vi "WaveFormGen.vi"(0 "电源干扰测试状态":refnum<vi>, 1 "开始测试":refnum<vi>, 2 "电池恢复波形参数":T4={"最低电压持续时间 2"=10, "最终电压 2"=12.0, "最低电压2"=7.5, "初始电压时间 2"=10, "初始电压2"=12.0, "恢复时间(s)"=600}, 5 "ACC点火波形参数":T5={"初始电压"=12.0, "初始电压时间"=500, "最低点电压"=7.5, "上升点电压"=10.0, "从最低点到上升点时间"=100.0, "波动电压持续时间"=200, "从上升点到最终点时间"=3000.0, "最终点电压"=12.0, "最低点持续时间"=20} {"从上升点到最终点时间" format="%#_13g"; "从最低点到上升点时间" format="%#_13g"}, 7 "电压瞬断波形参数":cluster{"电源电压":dbl, "周期(ms)":i32, "周期数":i32}={"电源电压"=14.0, "周期(ms)"=2, "周期数"=2} {"电源电压" format="%#_13g"}, 9 "电压缓变波形参数":T3={"最低电压持续时间 3"=1, "最高电压 3"=12.0, "最低电压2 2"=5.0, "初始电压时间 3"=1, "初始电压2 2"=12.0, "变化档位"=enum."1V/s", "周期数"=10}, 12 "+B电压开机参数":cluster{"+B电压":dbl, "持续时间(s)":i32}={"+B电压"=12.3, "持续时间(s)"=1} {"+B电压" format="%#_13g"}, 13 "测试项目":T1(ring), 14 "电源正弦纹波参数":T2={"频率1"=500.0, "幅度Vp"=4.0, "频率2"=20000.0, "频率3"=500.0, "电压Vs"=14.0, "周期数 3"=1} {"电压Vs" format="%#_13g"; "频率3" format="%#_13g"; "频率2" format="%#_13g"; "幅度Vp" format="%#_13g"; "频率1" format="%#_13g"}) -> (4 "waveform out":waveform(dbl))   [LabVIEW 2013]
uses:
  <vilib>/Analysis/1siggen.llb/Ramp Pattern by Samples.vi
  <vilib>/Waveform/WDTOps.llb/WDT Append Waveforms DBL.vi
  <vilib>/Analysis/NI_AALBase.lvlib
  <vilib>/measure/NI_MABase.lvlib
panel:
  # "(ms)"
  # "(ms)"
  # "(ms)"
  # "(ms)"
  # "(ms)"
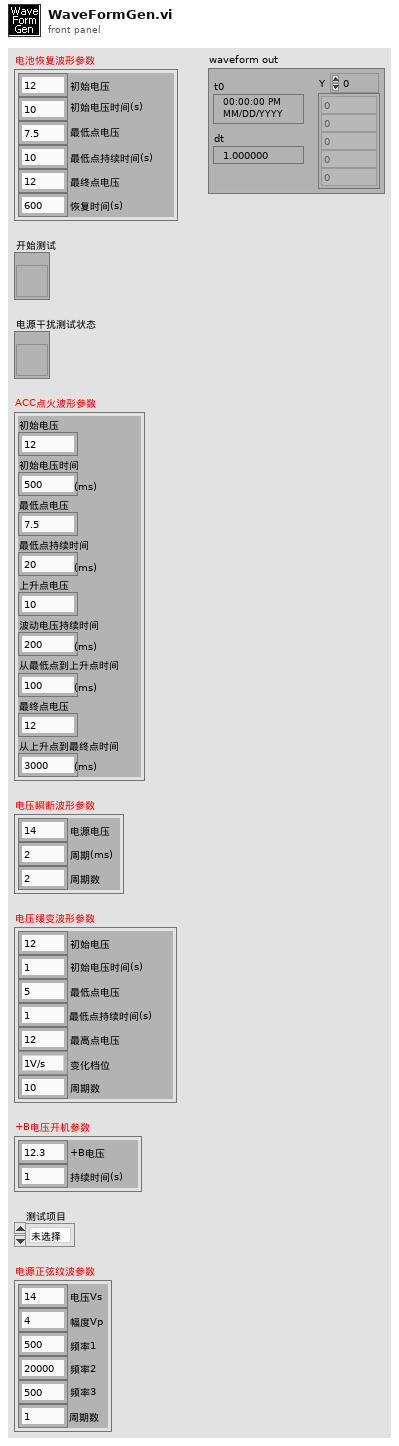
[diagram p1: front panel]
types:
  T1 = enum32{"未选择", "电源正弦纹波", "电压瞬断", "电池恢复", "电压缓变", "+B电压开机", "ACC点火"}
  T2 = cluster{"频率1":dbl, "幅度Vp":dbl, "频率2":dbl, "频率3":dbl, "电压Vs":dbl, "周期数 3":i32}
  T3 = cluster{"最低电压持续时间 3":i32, "最高电压 3":dbl, "最低电压2 2":dbl, "初始电压时间 3":i32, "初始电压2 2":dbl, "变化档位":enum16{"1V/s", "10V/s", "1V/min"}, "周期数":i32}
  T4 = cluster{"最低电压持续时间 2":i32, "最终电压 2":dbl, "最低电压2":dbl, "初始电压时间 2":i32, "初始电压2":dbl, "恢复时间(s)":i32}
  T5 = cluster{"初始电压":dbl, "初始电压时间":i32, "最低点电压":dbl, "上升点电压":dbl, "从最低点到上升点时间":dbl, "波动电压持续时间":i32, "从上升点到最终点时间":dbl, "最终点电压":dbl, "最低点持续时间":i32}
  T6 = enum8{"Enabled", "Disabled", "Disabled and Grayed Out"}
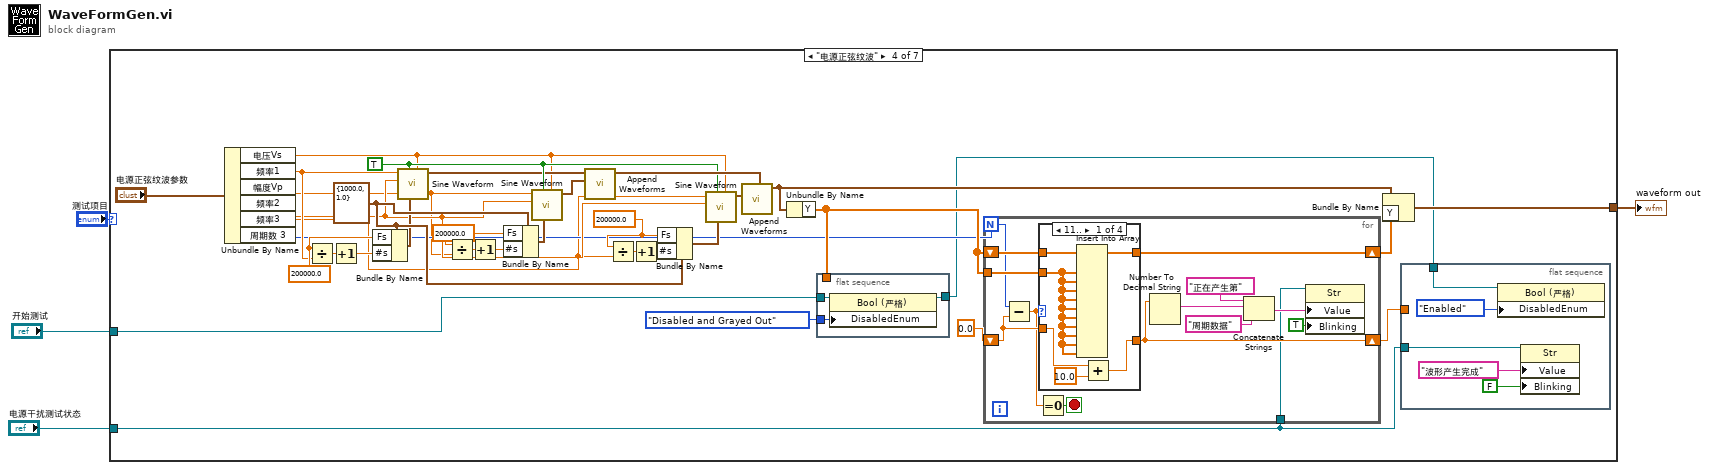
[diagram p0: block diagram]
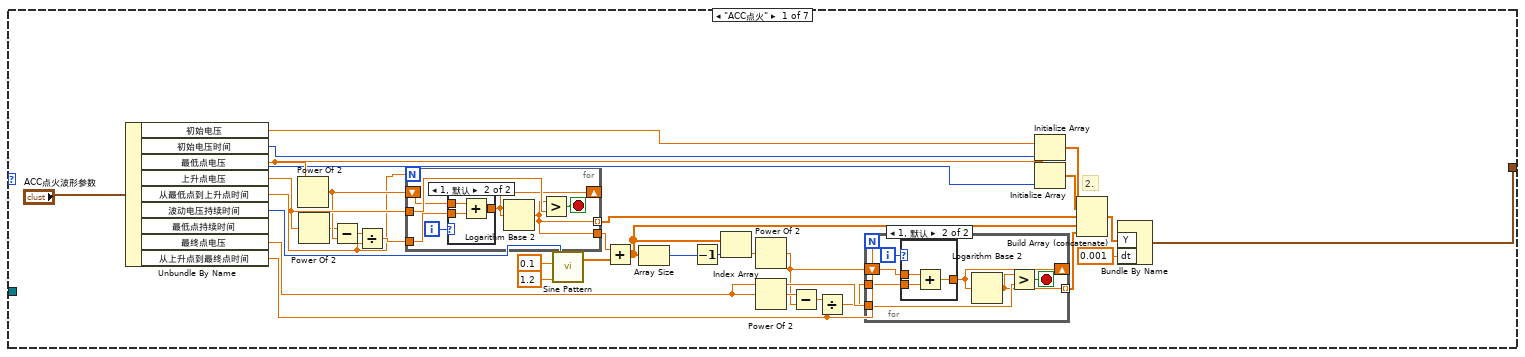
[diagram p2: hidden frame]
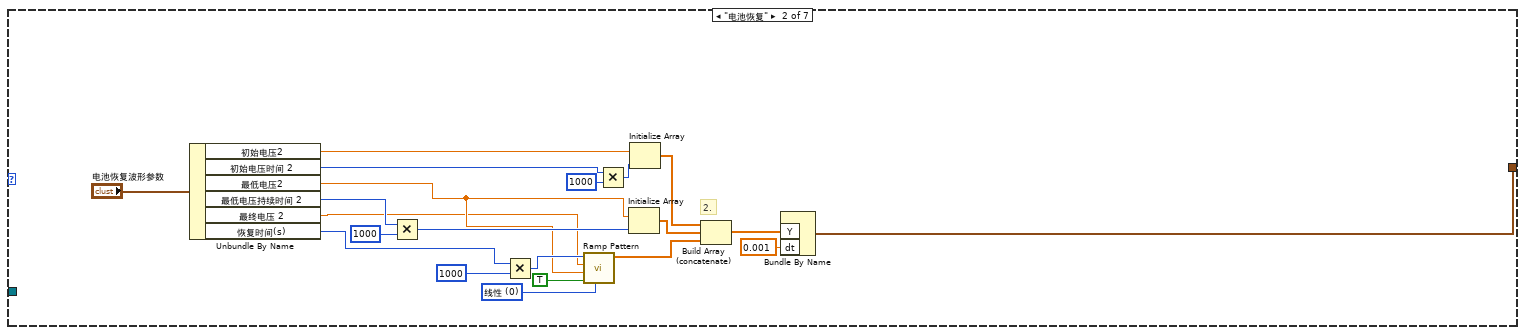
[diagram p5: hidden frame]
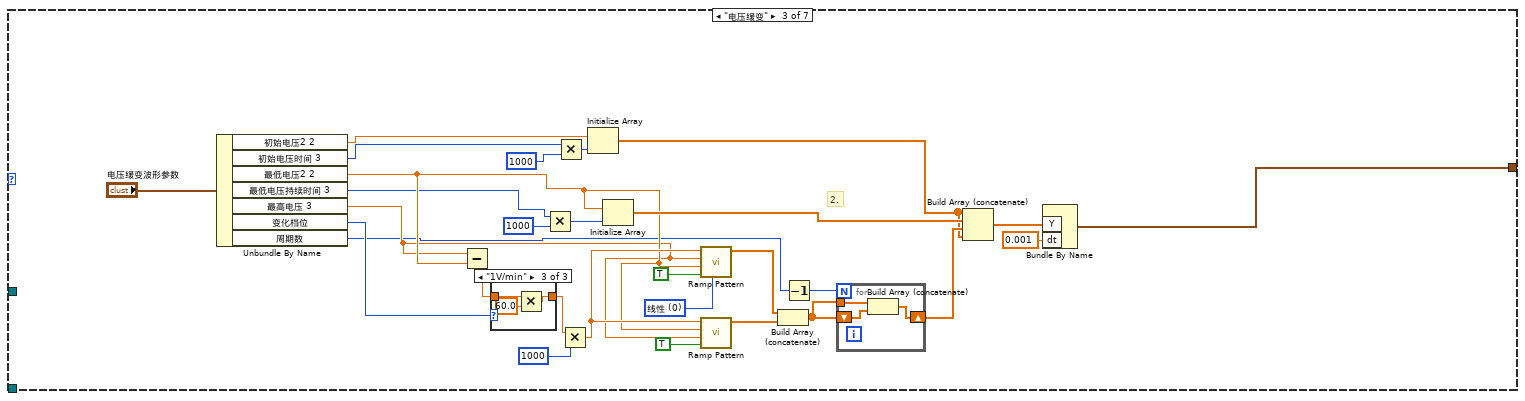
[diagram p6: hidden frame]
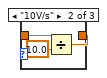
[diagram p8: hidden frame]
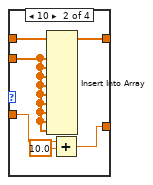
[diagram p9: hidden frame]
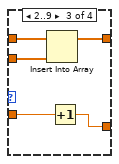
[diagram p10: hidden frame]
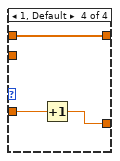
[diagram p11: hidden frame]
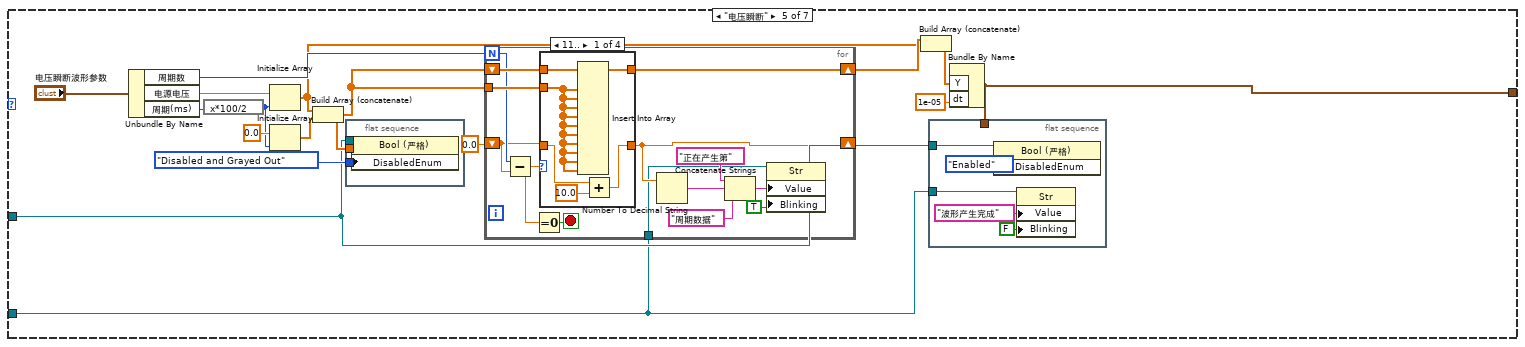
[diagram p12: hidden frame]
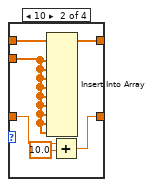
[diagram p13: hidden frame]
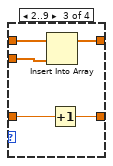
[diagram p14: hidden frame]
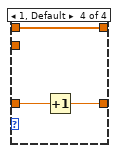
[diagram p15: hidden frame]
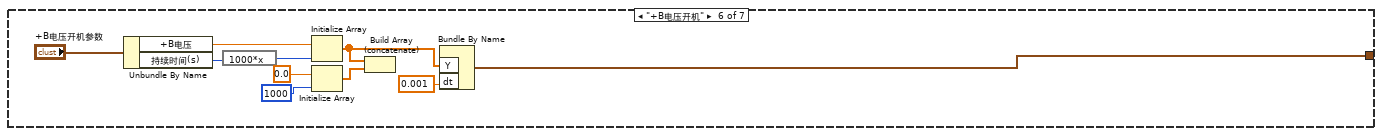
[diagram p16: hidden frame]
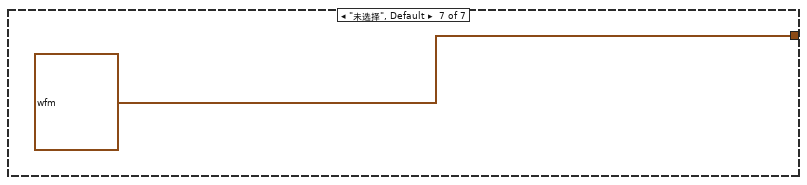
[diagram p17: hidden frame]
diagram:
  n1 = case shown="\"电源正弦纹波\"" "测试项目" {
    tunnel: [w10 w67 w90 w154 w199 w258 waveform(dbl) {"t0"=timestamp(0 s since 1904-01-01), "dt"=1.0, "Y"=[]} ("waveform out")] -> w3
    tunnel: "开始测试" -> [_ _ _ w122 w198 _ _]
    tunnel: "电源干扰测试状态" -> [_ _ _ w120 w197 _ _]
    frame "ACC点火" {
      # "2."
      n2 = Unbundle By Name("ACC点火波形参数") -> ("初始电压"=w34:dbl, "初始电压时间"=w6:i32, "最低点电压"=w35:dbl, "上升点电压"=w36:dbl, "从最低点到上升点时间"=w8:dbl, "波动电压持续时间"=w9:i32, "最低点持续时间"=w5:i32, "最终点电压"=w37:dbl, "从上升点到最终点时间"=w7:dbl)
      n3 = Power Of 2(x=w35) -> (2^x=w17:dbl)
      n4 = Power Of 2(x=w36) -> (2^x=w14:dbl)
      n5 = Subtract(x=w14, y=w17) -> (x-y=w15:dbl)
      n6 = Divide(x=w15, y=w8) -> (x/y=w16:dbl)
      n7 = for {
        N: w8 -> [_]
        tunnel: [w49] -> w32 mode=indexing
        tunnel: w36 -> [w54]
        shift-right: [w52] -> _
        shift-left: w17 -> [w53]
        tunnel: w16 -> [w51]
        tunnel: [w49] -> w30
        i -> [w50]
        stop <- w55 stop-if-true
        n8 = case shown="1, 默认" w50 {
          tunnel: w53 -> [w56 w59]
          tunnel: [w56 w58] -> w52
          tunnel: w51 -> [_ w57]
          frame 0 {
          }
          frame 1, Default {
            n9 = Add(x=w59, y=w57) -> (x+y=w58:dbl)
          }
        }
        n10 = Logarithm Base 2(1:w52) -> (0:w49:dbl)
        n11 = Greater?(x=w49, y=w54) -> (0:w55:bool)
      }
      n12 = call <vilib>:"Sine Pattern.vi"("cycles"=1.2, "amplitude"=0.1, "samples"=w9) -> ("Sinusoidal Pattern"=w24:dbl[])  [unwired: 1 in, 1 out]
      n13 = Add(x=w30, y=w24) -> (x+y=w29:dbl[])
      n14 = Array Size(array=w29) -> (size(s)=w25:i32)
      n15 = Decrement(x=w25) -> (x-1=w26:i32)
      n16 = Index Array(array=w29, index=w26) -> (element=w27:dbl)
      n17 = Power Of 2(x=w27) -> (2^x=w20:dbl)
      n18 = Power Of 2(x=w37) -> (2^x=w23:dbl)
      n19 = Subtract(x=w23, y=w20) -> (x-y=w22:dbl)
      n20 = Divide(x=w22, y=w7) -> (x/y=w21:dbl)
      n21 = for {
        N: w7 -> [_]
        tunnel: [w38] -> w28 mode=indexing
        tunnel: w37 -> [w43]
        shift-right: [w41] -> _
        shift-left: w20 -> [w42]
        tunnel: w21 -> [w40]
        i -> [w39]
        stop <- w44 stop-if-true
        n22 = case shown="1, 默认" w39 {
          tunnel: w42 -> [w45 w48]
          tunnel: [w45 w47] -> w41
          tunnel: w40 -> [_ w46]
          frame 0 {
          }
          frame 1, Default {
            n23 = Add(x=w48, y=w46) -> (x+y=w47:dbl)
          }
        }
        n24 = Logarithm Base 2(1:w41) -> (0:w38:dbl)
        n25 = Greater?(x=w38, y=w43) -> (0:w44:bool)
      }
      n26 = Initialize Array(w34, w6) -> (w11:dbl[])
      n27 = Initialize Array(w35, w5) -> (w31:dbl[])
      n28 = Build Array (concatenate)(w11, w31, w32, w29, w28) -> (w12:dbl[])
      n29 = Bundle By Name("Y"=w12, "dt"=0.001) -> (w10:waveform(dbl))  [unwired: 1 in]
    }
    frame "电池恢复" {
      w75 = u16 0 items=["线性", "对数"] ("type")
      # "2."
      n30 = Unbundle By Name("电池恢复波形参数") -> ("初始电压2"=w65:dbl, "初始电压时间 2"=w64:i32, "最低电压2"=w63:dbl, "最低电压持续时间 2"=w62:i32, "最终电压 2"=w61:dbl, "恢复时间(s)"=w60:i32)
      n31 = Multiply(x=w62, y=1000) -> (x*y=w70:i32)
      n32 = Multiply(x=w60, y=1000) -> (x*y=w68:i32)
      n33 = call-poly <vilib>:"Ramp Pattern.vi"("type"=w75, "exclude end?"=TRUE, "start"=w63, "end"=w61, "samples"=w68) -> ("Ramp Pattern"=w76:dbl[])  [unwired: 5 in, 1 out]
      n34 = Multiply(x=w64, y=1000) -> (x*y=w72:i32)
      n35 = Initialize Array(w63, w70) -> (w77:dbl[])
      n36 = Initialize Array(w65, w72) -> (w80:dbl[])
      n37 = Build Array (concatenate)(w80, w77, w76) -> (w79:dbl[])
      n38 = Bundle By Name("Y"=w79, "dt"=0.001) -> (w67:waveform(dbl))  [unwired: 1 in]
    }
    frame "电压缓变" {
      w106 = u16 0 items=["线性", "对数"] ("type")
      # "2."
      n39 = Unbundle By Name("电压缓变波形参数") -> ("初始电压2 2"=w88:dbl, "初始电压时间 3"=w87:i32, "最低电压2 2"=w86:dbl, "最低电压持续时间 3"=w85:i32, "最高电压 3"=w84:dbl, "变化档位"=w83:enum16{"1V/s", "10V/s", "1V/min"}, "周期数"=w82:i32)
      n40 = Subtract(x=w84, y=w86) -> (x-y=w99:dbl)
      n41 = case shown="\"1V/min\"" w83 {
        tunnel: w99 -> [w113 w116 w119]
        tunnel: [w113 w114 w117] -> w98
        frame "1V/s", Default {
        }
        frame "10V/s" {
          n42 = Divide(x=w116, y=10.0) -> (x/y=w114:dbl)
        }
        frame "1V/min" {
          n43 = Multiply(x=w119, y=60.0) -> (x*y=w117:dbl)
        }
      }
      n44 = Multiply(x=w85, y=1000) -> (x*y=w101:i32)
      n45 = Multiply(x=w87, y=1000) -> (x*y=w103:i32)
      n46 = Multiply(x=w98, y=1000) -> (x*y=w96:dbl)
      n47 = Initialize Array(w88, w103) -> (w81:dbl[])
      n48 = Initialize Array(w86, w101) -> (w107:dbl[])
      n49 = call-poly <vilib>:"Ramp Pattern.vi"("type"=w106, "exclude end?"=TRUE, "start"=w86, "end"=w84, "samples"=w96) -> ("Ramp Pattern"=w95:dbl[])  [unwired: 5 in, 1 out]
      n50 = call-poly <vilib>:"Ramp Pattern.vi"("exclude end?"=TRUE, "start"=w84, "end"=w86, "samples"=w96) -> ("Ramp Pattern"=w94:dbl[])  [unwired: 6 in, 1 out]
      n51 = Build Array (concatenate)(w95, w94) -> (w92:dbl[])
      n52 = Decrement(x=w82) -> (x-1=w91:i32)
      n53 = for {
        N: w91 -> [_]
        shift-right: [w110] -> w93
        shift-left: w92 -> [w112]
        tunnel: w92 -> [w111]
        n54 = Build Array (concatenate)(w111, w112) -> (w110:dbl[])
      }
      n55 = Build Array (concatenate)(w81, w107, w93, w81) -> (w109:dbl[])
      n56 = Bundle By Name("Y"=w109, "dt"=0.001) -> (w90:waveform(dbl))  [unwired: 1 in]
    }
    frame "电源正弦纹波" {
      w141 = 200000.0 ("Fs")
      w140 = 200000.0 ("Fs")
      w135 = 200000.0 ("Fs")
      w146 = TRUE ("reset signal")
      w145 = cluster{"Fs":dbl, "#s":dbl} {"Fs"=1000.0, "#s"=1.0} ("sampling info")
      n57 = Unbundle By Name("电源正弦纹波参数") -> ("电压Vs"=w129:dbl, "频率1"=w128:dbl, "幅度Vp"=w127:dbl, "频率2"=w124:dbl, "频率3"=w125:dbl, "周期数 3"=w126:i32)
      n58 = Divide(x=w135, y=w128) -> (x/y=w136:dbl)
      n59 = Increment(x=w136) -> (x+1=w137:dbl)
      n60 = Bundle By Name(cluster=w145, "Fs"=w135, "#s"=w137) -> (w131:cluster{"Fs":dbl, "#s":dbl})
      n61 = call <vilib>:"Sine Waveform.vi"("offset"=w129, "sampling info"=w131, "reset signal"=w146, "amplitude"=w127, "frequency"=w128) -> ("signal out"=w134:waveform(dbl))  [unwired: 5 in, 1 out]
      n62 = Divide(x=w140, y=w124) -> (x/y=w138:dbl)
      n63 = Increment(x=w138) -> (x+1=w139:dbl)
      n64 = Bundle By Name(cluster=w145, "Fs"=w140, "#s"=w139) -> (w132:cluster{"Fs":dbl, "#s":dbl})
      n65 = call <vilib>:"Sine Waveform.vi"("offset"=w129, "sampling info"=w132, "reset signal"=w146, "amplitude"=w127, "frequency"=w124) -> ("signal out"=w133:waveform(dbl))  [unwired: 5 in, 1 out]
      n66 = call-poly <vilib>:"Append Waveforms.vi"("waveform B"=w133, "waveform A"=w134) -> ("waveform out"=w147:waveform(dbl))  [unwired: 8 in, 1 out]
      n67 = Divide(x=w141, y=w125) -> (x/y=w143:dbl)
      n68 = Increment(x=w143) -> (x+1=w142:dbl)
      n69 = Bundle By Name(cluster=w145, "Fs"=w141, "#s"=w142) -> (w144:cluster{"Fs":dbl, "#s":dbl})
      n70 = call <vilib>:"Sine Waveform.vi"("offset"=w129, "sampling info"=w144, "reset signal"=w146, "amplitude"=w127, "frequency"=w125) -> ("signal out"=w148:waveform(dbl))  [unwired: 5 in, 1 out]
      n71 = call-poly <vilib>:"Append Waveforms.vi"("waveform B"=w148, "waveform A"=w147) -> ("waveform out"=w123:waveform(dbl))  [unwired: 8 in, 1 out]
      n72 = Unbundle By Name(w123) -> ("Y"=w152:dbl[])
      n73 = flat-sequence {
        tunnel: T6."Disabled and Grayed Out" ("禁用") -> [w162]
        tunnel: w152 -> [_]
        tunnel: w122 -> [w161]
        tunnel: [w160] -> w121
        frame #0 {
          n74 = property on="属性节点" class="Bool (严格)"(reference=w161, "DisabledEnum"=w162) -> (reference out=w160:refnum<vi>)  [unwired: 1 in, 1 out]
        }
      }
      n75 = for {
        N: w126 -> [w168]
        shift-right: [w176] -> w150
        shift-left: w152 -> [w175]
        tunnel: w152 -> [w169]
        shift-right: [w164] -> w153
        shift-left: 0.0 -> [w167]
        tunnel: w120 -> [w163]
        stop <- w165 stop-if-true
        n76 = Subtract(x=w168, y=w167) -> (x-y=w166:dbl)
        n77 = Equal To 0?(x=w166) -> (x = 0?=w165:bool)
        n78 = case shown="11.." w166 {
          tunnel: [w182 w188 w193 w196] -> w176
          tunnel: w175 -> [w181 w187 w192 w196]
          tunnel: w169 -> [w177 w183 w191 _]
          tunnel: [w180 w186 w190 w194] -> w164
          tunnel: w167 -> [w179 w185 w189 w195]
          frame 11.. {
            n79 = Insert Into Array(array=w181, new element #1=w177, new element #2=w177, new element #3=w177, new element #4=w177, new element #5=w177, new element #6=w177, new element #7=w177, new element #8=w177, new element #9=w177, new element #10=w177) -> (w182:dbl[])  [unwired: 1 in]
            n80 = Add(x=w179, y=10.0) -> (x+y=w180:dbl)
          }
          frame 10 {
            n81 = Insert Into Array(array=w187, new element #1=w183, new element #2=w183, new element #3=w183, new element #4=w183, new element #5=w183, new element #6=w183, new element #7=w183, new element #8=w183, new element #9=w183) -> (w188:dbl[])  [unwired: 1 in]
            n82 = Add(x=w185, y=10.0) -> (x+y=w186:dbl)
          }
          frame 2..9 {
            n83 = Insert Into Array(array=w192, new element=w191) -> (w193:dbl[])  [unwired: 1 in]
            n84 = Increment(x=w189) -> (x+1=w190:dbl)
          }
          frame 1, Default {
            n85 = Increment(x=w195) -> (x+1=w194:dbl)
          }
        }
        n86 = Number To Decimal String(number=w164) -> (decimal integer string=w172:string)  [unwired: 1 in]
        n87 = Concatenate Strings("正在产生第" ("字符串"), w172, "周期数据" ("字符串")) -> (w173:string)
        n88 = property on="属性节点" class="Str"(reference=w163, "Value"=w173, "Blinking"=TRUE ("闪烁")) -> ()  [unwired: 1 in, 2 out]
      }
      n89 = Bundle By Name(cluster=w123, "Y"=w150) -> (w154:waveform(dbl))
      n90 = flat-sequence {
        tunnel: w153 -> [_]
        tunnel: w120 -> [w156]
        tunnel: w121 -> [w155]
        frame #0 {
          n91 = property on="属性节点" class="Bool (严格)"(reference=w155, "DisabledEnum"=T6."Enabled" ("禁用")) -> ()  [unwired: 1 in, 2 out]
          n92 = property on="属性节点" class="Str"(reference=w156, "Value"="波形产生完成" ("测试状态"), "Blinking"=FALSE ("闪烁")) -> ()  [unwired: 1 in, 2 out]
        }
      }
    }
    frame "电压瞬断" {
      n93 = Unbundle By Name("电压瞬断波形参数") -> ("周期数"=w205:i32, "电源电压"=w204:dbl, "周期(ms)"=w203:i32)
      n94 = expression code="x*100/2"(w203) -> (w208:i32)
      n95 = Initialize Array(w204, w208) -> (w201:dbl[])
      n96 = Initialize Array(0.0 ("元素"), w208) -> (w212:dbl[])
      n97 = Build Array (concatenate)(w201, w212) -> (w209:dbl[])
      n98 = flat-sequence {
        tunnel: w209 -> [_]
        tunnel: T6."Disabled and Grayed Out" ("禁用") -> [w220]
        tunnel: w198 -> [w219]
        frame #0 {
          n99 = property on="属性节点" class="Bool (严格)"(reference=w219, "DisabledEnum"=w220) -> ()  [unwired: 1 in, 2 out]
        }
      }
      n100 = for {
        N: w205 -> [w226]
        shift-right: [w234] -> w202
        shift-left: w209 -> [w233]
        tunnel: w209 -> [w227]
        shift-right: [w222] -> _
        shift-left: 0.0 -> [w225]
        tunnel: w197 -> [w221]
        stop <- w223 stop-if-true
        n101 = Subtract(x=w226, y=w225) -> (x-y=w224:dbl)
        n102 = Equal To 0?(x=w224) -> (x = 0?=w223:bool)
        n103 = case shown="11.." w224 {
          tunnel: [w240 w246 w251 w254] -> w234
          tunnel: w233 -> [w239 w245 w250 w254]
          tunnel: w227 -> [w235 w241 w249 _]
          tunnel: [w238 w244 w248 w252] -> w222
          tunnel: w225 -> [w237 w243 w247 w253]
          frame 11.. {
            n104 = Insert Into Array(array=w239, new element #1=w235, new element #2=w235, new element #3=w235, new element #4=w235, new element #5=w235, new element #6=w235, new element #7=w235, new element #8=w235, new element #9=w235, new element #10=w235) -> (w240:dbl[])  [unwired: 1 in]
            n105 = Add(x=w237, y=10.0) -> (x+y=w238:dbl)
          }
          frame 10 {
            n106 = Insert Into Array(array=w245, new element #1=w241, new element #2=w241, new element #3=w241, new element #4=w241, new element #5=w241, new element #6=w241, new element #7=w241, new element #8=w241, new element #9=w241) -> (w246:dbl[])  [unwired: 1 in]
            n107 = Add(x=w243, y=10.0) -> (x+y=w244:dbl)
          }
          frame 2..9 {
            n108 = Insert Into Array(array=w250, new element=w249) -> (w251:dbl[])  [unwired: 1 in]
            n109 = Increment(x=w247) -> (x+1=w248:dbl)
          }
          frame 1, Default {
            n110 = Increment(x=w253) -> (x+1=w252:dbl)
          }
        }
        n111 = Number To Decimal String(number=w222) -> (decimal integer string=w230:string)  [unwired: 1 in]
        n112 = Concatenate Strings("正在产生第" ("字符串"), w230, "周期数据" ("字符串")) -> (w231:string)
        n113 = property on="属性节点" class="Str"(reference=w221, "Value"=w231, "Blinking"=TRUE ("闪烁")) -> ()  [unwired: 1 in, 2 out]
      }
      n114 = Build Array (concatenate)(w202, w201) -> (w200:dbl[])
      n115 = flat-sequence {
        tunnel: w199 -> [_]
        tunnel: w197 -> [w215]
        tunnel: w198 -> [w214]
        frame #0 {
          n116 = property on="属性节点" class="Bool (严格)"(reference=w214, "DisabledEnum"=T6."Enabled" ("禁用")) -> ()  [unwired: 1 in, 2 out]
          n117 = property on="属性节点" class="Str"(reference=w215, "Value"="波形产生完成" ("测试状态"), "Blinking"=FALSE ("闪烁")) -> ()  [unwired: 1 in, 2 out]
        }
      }
      n118 = Bundle By Name("Y"=w200, "dt"=1e-05) -> (w199:waveform(dbl))  [unwired: 1 in]
    }
    frame "+B电压开机" {
      n119 = Unbundle By Name("+B电压开机参数") -> ("+B电压"=w255:dbl, "持续时间(s)"=w256:i32)
      n120 = expression code="1000*x"(w256) -> (w261:i32)
      n121 = Initialize Array(w255, w261) -> (w259:dbl[])
      n122 = Initialize Array(0.0 ("元素"), 1000 ("维数大小")) -> (w263:dbl[])
      n123 = Build Array (concatenate)(w259, w263) -> ()  [unwired: 1 out]
      n124 = Bundle By Name("Y"=w259, "dt"=0.001) -> (w258:waveform(dbl))  [unwired: 1 in]
    }
    frame "未选择", Default {
    }
  }
  "waveform out" <- w3
